vi "LV SciSDK INIT CUSTOM PACKET.vi"(0 "Custom Packet Name":string, 1 "High Performance":string(combo)="false", 2 "Acq Mode":string(combo)="blocking", 3 "Thread":string(combo)="false", 4 "Handle In":T2, 5 "error in (no error)":errorcluster, 6 "Check Align Word":string(combo)="false", 8 "Timeout":i32=100, 10 "Acq Len":u32=1024, 12 "Threaded Buffer Size":u32=100000) -> (18 "CP Handle Out":T1, 19 "error out":errorcluster)   [LabVIEW 2021]
uses:
  SciSDK_Labview.lvlib
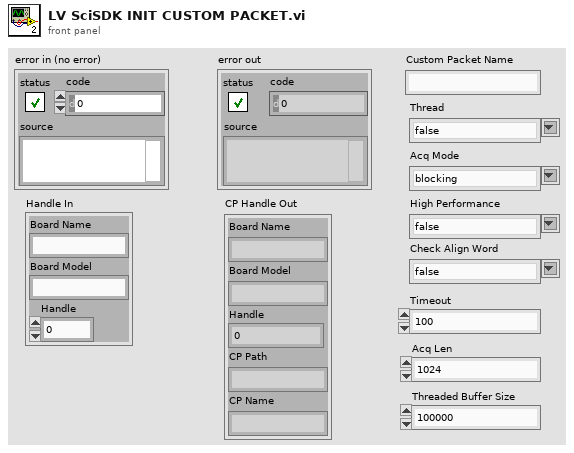
[diagram p1: front panel]
types:
  T1 = cluster{"Board Name":string, "Board Model":string, "Handle":u64, "CP Path":string, "CP Name":string}
  T2 = cluster{"Board Name":string, "Board Model":string, "Handle":u64}
  T3 = cluster{"Board Name":string, "Board Model":string, "Handle":u64, string, "Custom Packet Name":string}
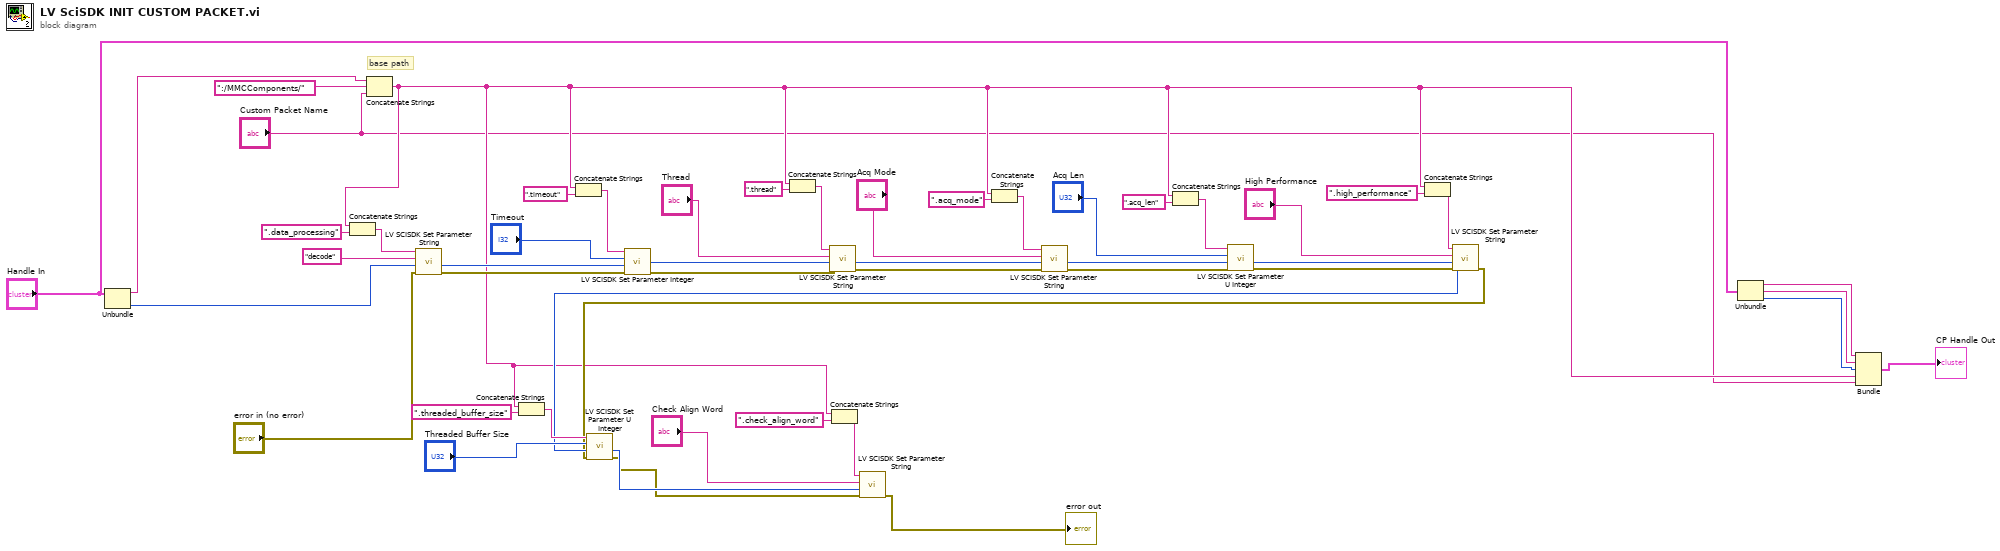
[diagram p0: block diagram]
diagram:
  # "base path"
  n1 = Unbundle("Handle In") -> ("Board Name"=w45:string, "Handle"=w40:u64)  [unwired: 1 out]
  n2 = Concatenate Strings(w45, ":/MMCComponents/" ("string"), "Custom Packet Name") -> (w2:string)
  n3 = Concatenate Strings(w2, ".data_processing" ("string")) -> (w42:string)
  n4 = call "LV SCISDK Set Parameter String.vi"("error in (no error)"="error in (no error)", "handle"=w40, "value"="decode", "Path"=w42) -> ("error out"=w26:errorcluster, "handle out"=w37:u64)  [unwired: 5 in, 1 out]
  n5 = Concatenate Strings(w2, ".threaded_buffer_size" ("string")) -> (w12:string)
  n6 = Concatenate Strings(w2, ".timeout" ("string")) -> (w35:string)
  n7 = call "LV SCISDK Set Parameter Integer.vi"("error in (no error)"=w26, "handle"=w37, "value"="Timeout", "Path"=w35) -> ("error out"=w25:errorcluster, "handle out"=w27:u64)  [unwired: 5 in, 1 out]
  n8 = Concatenate Strings(w2, ".thread" ("string")) -> (w33:string)
  n9 = call "LV SCISDK Set Parameter String.vi"("error in (no error)"=w25, "handle"=w27, "value"="Thread", "Path"=w33) -> ("error out"=w24:errorcluster, "handle out"=w28:u64)  [unwired: 5 in, 1 out]
  n10 = Concatenate Strings(w2, ".check_align_word" ("string")) -> (w6:string)
  n11 = Concatenate Strings(w2, ".acq_mode" ("string")) -> (w31:string)
  n12 = call "LV SCISDK Set Parameter String.vi"("error in (no error)"=w24, "handle"=w28, "value"="Acq Mode", "Path"=w31) -> ("error out"=w23:errorcluster, "handle out"=w22:u64)  [unwired: 5 in, 1 out]
  n13 = Concatenate Strings(w2, ".acq_len" ("string")) -> (w20:string)
  n14 = call "LV SCISDK Set Parameter U Integer.vi"("error in (no error)"=w23, "handle"=w22, "value"="Acq Len", "Path"=w20) -> ("error out"=w17:errorcluster, "handle out"=w16:u64)  [unwired: 5 in, 1 out]
  n15 = Concatenate Strings(w2, ".high_performance" ("string")) -> (w14:string)
  n16 = call "LV SCISDK Set Parameter String.vi"("error in (no error)"=w17, "handle"=w16, "value"="High Performance", "Path"=w14) -> ("error out"=w9:errorcluster, "handle out"=w10:u64)  [unwired: 5 in, 1 out]
  n17 = call "LV SCISDK Set Parameter U Integer.vi"("error in (no error)"=w9, "handle"=w10, "value"="Threaded Buffer Size", "Path"=w12) -> ("error out"=w4:errorcluster, "handle out"=w5:u64)  [unwired: 5 in, 1 out]
  n18 = call "LV SCISDK Set Parameter String.vi"("error in (no error)"=w4, "handle"=w5, "value"="Check Align Word", "Path"=w6) -> ("error out"=→"error out":errorcluster)  [unwired: 5 in, 2 out]
  n19 = Unbundle("Handle In") -> ("Board Name"=w48:string, "Board Model"=w47:string, "Handle"=w46:u64)
  n20 = Bundle("Board Name"=w48, "Board Model"=w47, "Handle"=w46, w2, "Custom Packet Name"="Custom Packet Name") -> (→"CP Handle Out":T3)  [unwired: 1 in]
